vi "生成指令数组.vi"(0 "指令参数输入":T3) -> (1 "测试指令1":T1, 2 "测试指令2":T2, 3 "数组":string[](array[string]), 4 "数值":i32)   [LabVIEW 2015]
panel:
  # "TER   TCP  UDP  SMS"
  # "TER   TCP  UDP  SMS"
  # "TER   TCP  UDP  SMS"
  # "TER   TCP  UDP  SMS"
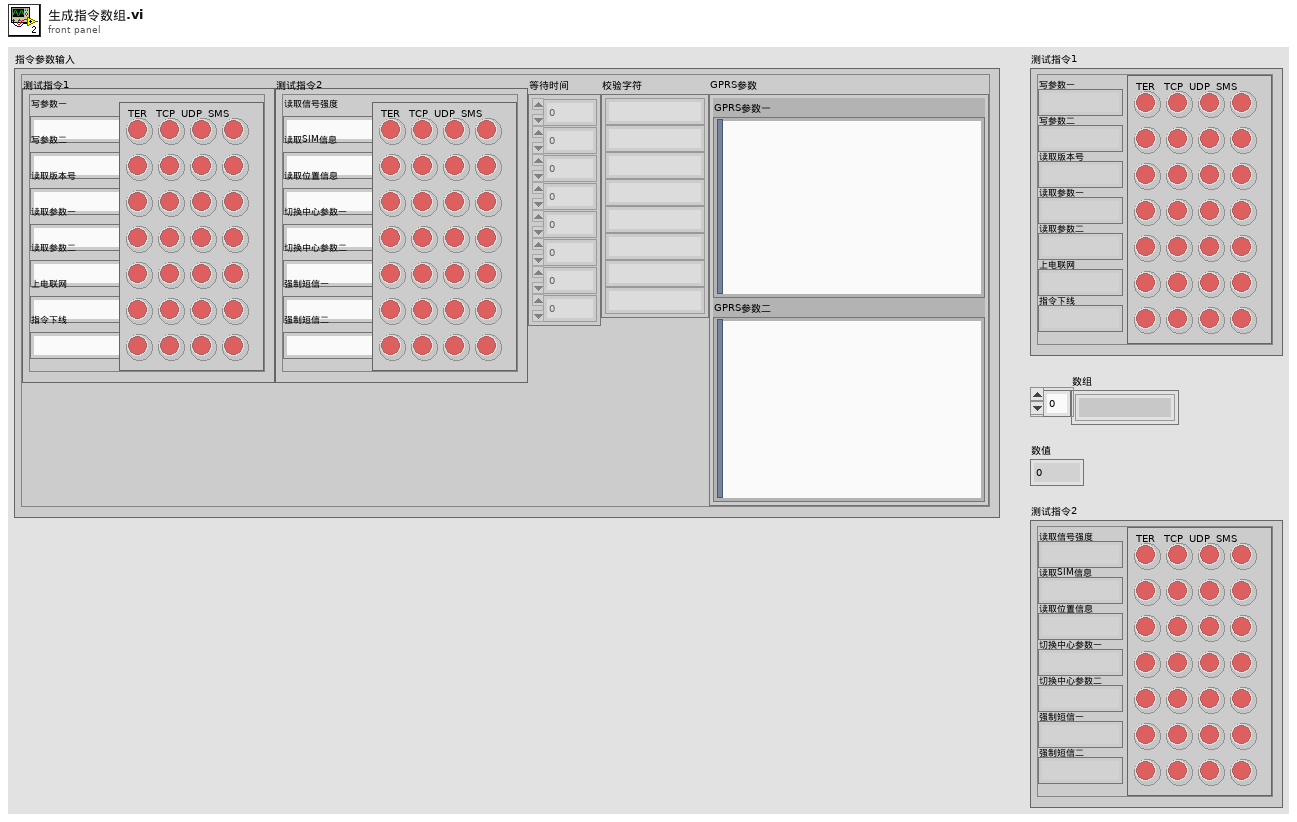
[diagram p1: front panel]
types:
  T1 = typedef "指令参数1.ctl" = cluster{"写参数一":string, "写参数二":string, "读取版本号":string, "读取参数一":string, "读取参数二":string, "上电联网":string, "指令下线":string, "指示灯":bool[][]}
  T2 = typedef "指令参数2.ctl" = cluster{"读取信号强度":string, "读取SIM信息":string, "读取位置信息":string, "切换中心参数一":string, "切换中心参数二":string, "强制短信一":string, "强制短信二":string, "指示灯":bool[][]}
  T3 = typedef "初始化测试指令.ctl" = cluster{"测试指令1":T1, "测试指令2":T2, "等待时间":u32[], "校验字符":string[], "GPRS参数":T4}
  T4 = typedef "GPRS参数.ctl" = cluster{"GPRS参数一":string, "GPRS参数二":string}
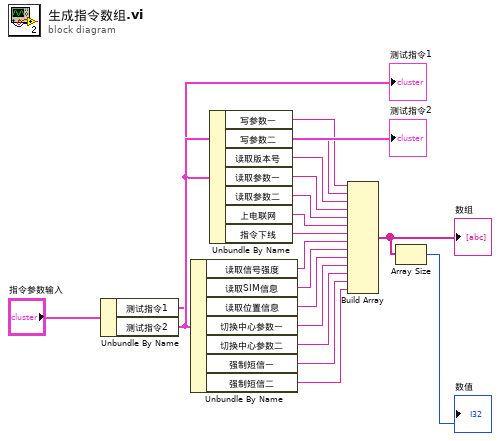
[diagram p0: block diagram]
diagram:
  n1 = Unbundle By Name("指令参数输入") -> ("测试指令1"=w17:T1, "测试指令2"=w18:T2)
  "测试指令2" <- w18
  "测试指令1" <- w17
  n2 = Unbundle By Name(w18) -> ("读取信号强度"=w9:string, "读取SIM信息"=w8:string, "读取位置信息"=w7:string, "切换中心参数一"=w6:string, "切换中心参数二"=w5:string, "强制短信一"=w4:string, "强制短信二"=w3:string)
  n3 = Unbundle By Name(w17) -> ("写参数一"=w16:string, "写参数二"=w15:string, "读取版本号"=w14:string, "读取参数一"=w13:string, "读取参数二"=w12:string, "上电联网"=w11:string, "指令下线"=w10:string)
  n4 = Build Array(w16, w15, w14, w13, w12, w11, w10, w9, w8, w7, w6, w5, w4, w3) -> (w2:string[])
  "数组" <- w2
  n5 = Array Size(array=w2) -> (size(s)=→"数值":i32)
